vi "ADI_IMU_ADIS16448_AHRS_RoboBees.vi"(8 "Yaw Axis":enum16{"X", "Y", "Z"}(ring)=enum."Z", 9 "Delta t":dbl, 10 "IMU Rates":dbl[](array[numeric])) -> (0 "Yaw":dbl(knob) scale=-180.0..180.0, 1 "Roll":dbl(knob) scale=-180.0..180.0, 2 "Pitch":dbl(knob) scale=-90.0..90.0, 3 "Output":cluster{"Pitch":dbl, "Roll":dbl, "Yaw":dbl})   [LabVIEW 2018, in "ADIS16448_IMU.lvlib"]
uses:
  ADIS16448_IMU.lvlib
panel:
  in  "Tilt Comp (Yaw)":bool=TRUE
  in  "tau mag":dbl=0.04
  in  "tau acc":dbl=0.95
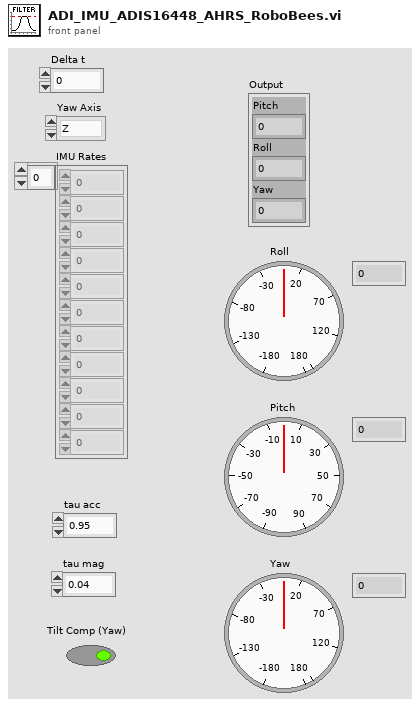
[diagram p1: front panel]
types:
  T1 = cluster{"Xaccel":dbl, "Yaccel":dbl, "Zaccel":dbl}
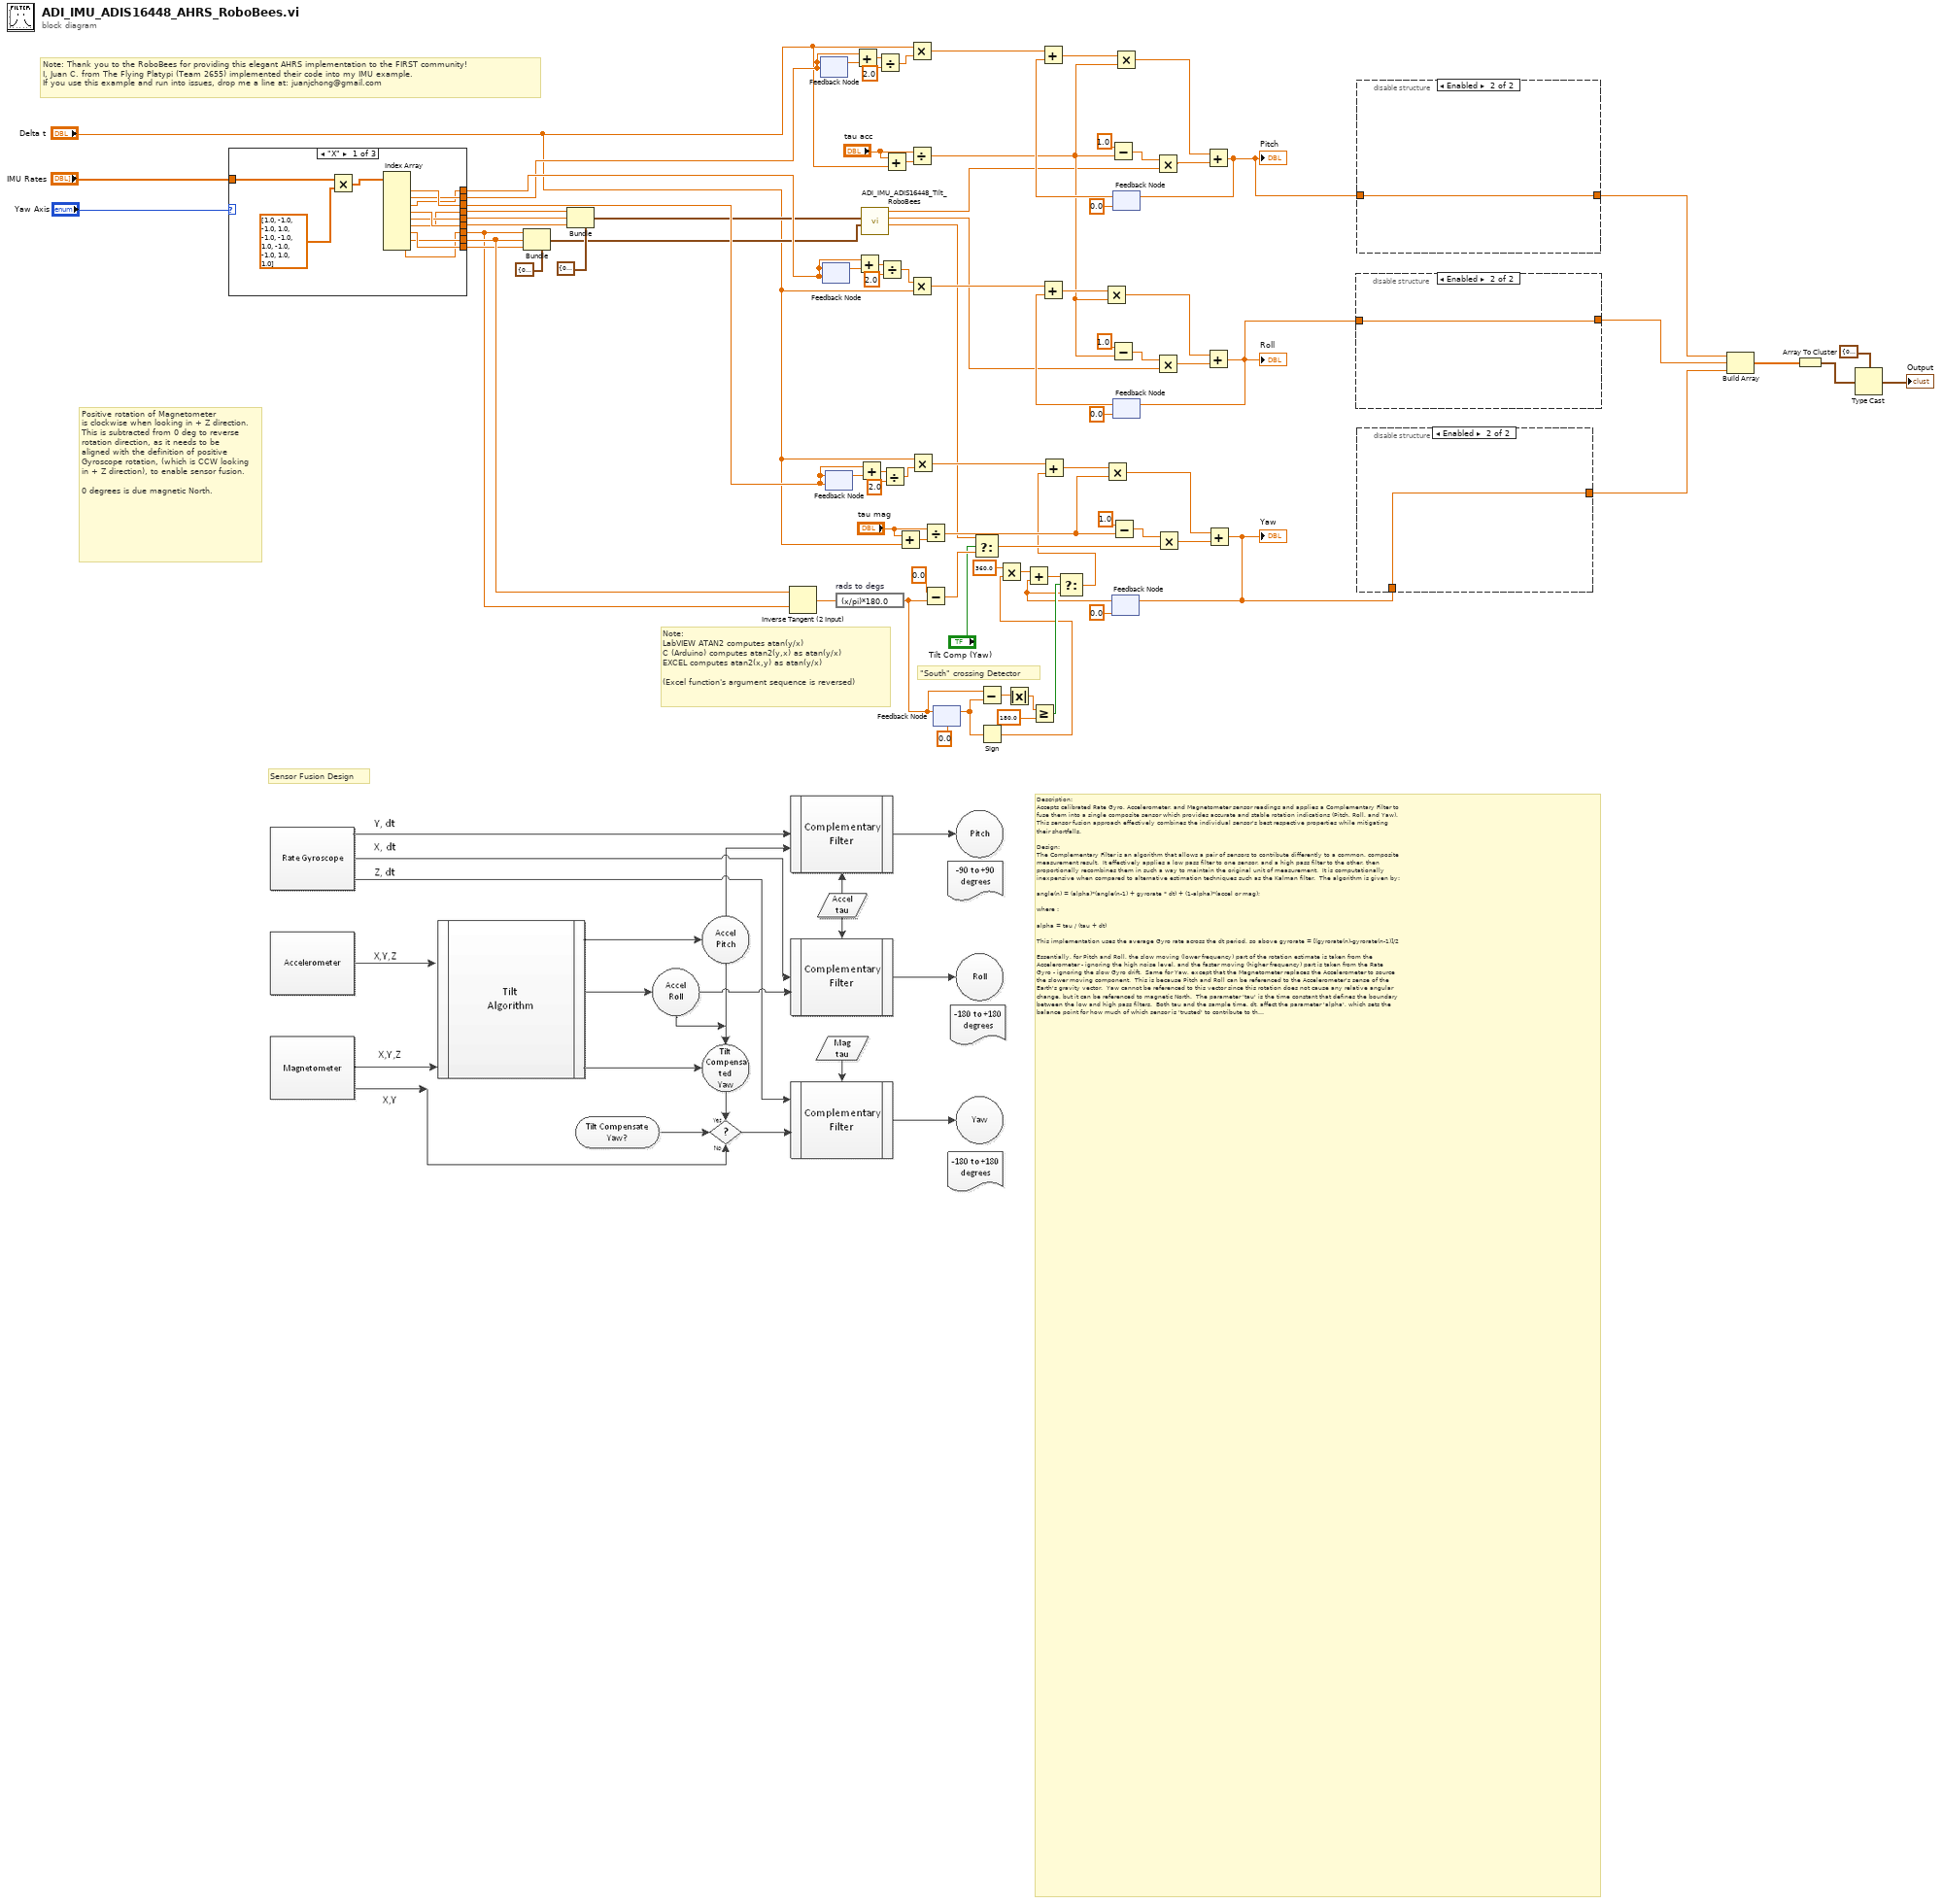
[diagram p0: block diagram]
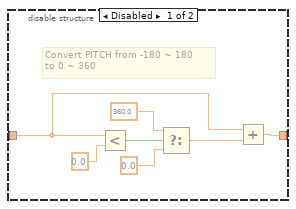
[diagram p2: hidden frame]
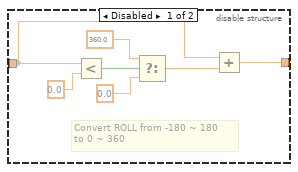
[diagram p3: hidden frame]
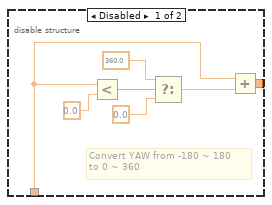
[diagram p4: hidden frame]
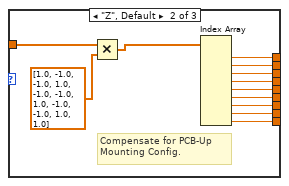
[diagram p5: hidden frame]
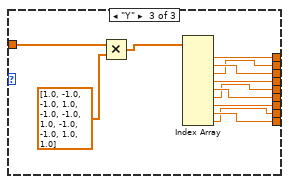
[diagram p6: hidden frame]
diagram:
  # "Note: Thank you to the RoboBees for providing this elegant AHRS implementation to the FIRST community!\nI, Juan C. from The Flying Platypi (Team 2655) implemented their code into my IMU example.\nIf you use this example and run into issues, drop me a line at: juanjchong@gmail.com"
  # "Sensor Fusion Design"
  # "Description:\nAccepts calibrated Rate Gyro, Accelerometer, and Magnetometer sensor readings and applies a Complementary Filter to\nfuse them into a single composite sensor which provides accurate and stable rotation indications (Pitch, Roll, and Yaw).\nThis sensor fusion approach effectively combines the individual sensor's best respective properties while mitigating\ntheir shortfalls.\n\nDesign:\nThe Complementary Filter is an algorithm that allows a pair of sensors to contribute differently to a common, composite\nmeasurement result.  It effectively applies a low pass filter to one sensor, and a high pass filter to the other, then\nproportionally recombines them in such a way to maintain the original unit of measurement.  It is computationally\ninexpensive when compared to alternative estimation techniques such as the Kalman filter.  The algorithm is given by:\n\nangle(n) = (alpha)*(angle(n-1) + gyrorate * dt) + (1-alpha)*(accel or mag);\n\nwhere : \n\nalpha = tau / (tau + dt)\n\nThis implementation uses the average Gyro rate across the dt period, so above gyrorate = [(gyrorate(n)-gyrorate(n-1)]/2\n\nEssentially, for Pitch and Roll, the slow moving (lower frequency) part of the rotation estimate is taken from the\nAccelerometer - ignoring the high noise level, and the faster moving (higher frequency) part is taken from the Rate \nGyro - ignoring the slow Gyro drift.  Same for Yaw, except that the Magnetometer replaces the Accelerometer to source\nthe slower moving component.  This is because Pitch and Roll can be referenced to the Accelerometer's sense of the\nEarth's gravity vector.  Yaw cannot be referenced to this vector since this rotation does not cause any relative angular\nchange, but it can be referenced to magnetic North.  The parameter 'tau' is the time constant that defines the boundary\nbetween the low and high pass filters.  Both tau and the sample time, dt, affect the parameter 'alpha', which sets the\nbalance point for how much of which sensor is 'trusted' to contribute to the rotation estimate.\n\nThe Complementary Filter algorithm is applied to each X/Y/Z rotation axis to compute R/P/Y outputs, respectively.\n\nMagnetometer readings are tilt-compensated when Tilt-Comp-(Yaw) is asserted (True), by the IMU TILT subVI.  This\ncreates what is known as a tilt-compensated compass, which allows Yaw to be insensitive to the effects of a\nnon-level sensor, but generates error in Yaw during movement (coordinate acceleration).\n\nThe Yaw \"South\" crossing detector is necessary to allow a smooth transition across the +/- 180 deg discontinuity (inherent\nin the ATAN function).  Since -180 deg is congruent with +180 deg, Yaw needs to jump between these values when\ncrossing South (North is 0 deg).  The design depends upon comparison of successive Yaw readings to detect a cross-over\nevent.  The cross-over detector monitors the current reading and evaluates how far it is from the previous reading.  If it\nis greater than the previous reading by the Discriminant (= 180 deg), then Yaw just crossed South.\n\nBy choosing 180 as the Discriminant, the only way the detector can produce a false positive, assuming a loop iteration\nof 70 msec, is for it to rotate >2,571 dps ... (2,571=180/.07).  This is faster than the ST L3GD20 Gyro can register.  The\ndetector produces a Boolean True upon detecting a South crossing.  This is used to alter the (n-1) Yaw which was\npreviously stored, either adding or subtracting 360 degrees as required to place the previous Yaw in the correct quadrant\nwhenever crossing occurs.  The Modulus function cannot be used here as the Complementary Filter algorithm has 'state'\n(needs to remember previous Yaw).\n \nWe are in effect stitching together two ends of a ruler for 'modular arithmetic' (clock math).\n\nInputs:\nGYRO - Gyro rate and sample time measurements.\nACCEL - Acceleration measurements.\nMAG - Magnetic measurements.\nTAU ACC - tau parameter used to set sensor balance between Accel and Gyro for Roll and Pitch.\nTAU MAG -  tau parameter used to set sensor balance between Mag and Gyro for Yaw.\nTILT COMP (Yaw) - Enables Yaw tilt-compensation if True.\n\nOutputs:\nROLL - Filtered Roll about sensor X-axis.\nPITCH - Filtered Pitch about sensor Y-axis.\nYAW - Filtered Yaw about sensor Z-axis.\n\nVI Properties:\nExecution Reentrancy is set to Non Reentrant Execution\n\nImplementation:\nIt's best to establish the optimum loop sample time first.  See IMU READ implementation notes for guidance.  Each\ntau parameter should then be adjusted to achieve optimum sensor fusion.  tau acc affects Roll and Pitch, tau mag affects\nYaw.  Start at value 1 or 2 and decrease by half each time until the result doesn't drift, but not so far that the result gets\nnoisy.  An optimum tau for this IMU is likely in the range of 1.0 to 0.01, for a loop sample time between 10 and 100 ms.\n\nNote that both sample timing (dt) and tau both affect the balance parameter, 'alpha'.  Adjusting either dt or tau will\nrequire the other to be readjusted to maintain a particular filter performance.\n\nIt is likely best to set Yaw tilt-compensation to off (False) if the Yaw value is to be used as feedback in a closed loop\ncontrol application.  The tradeoff is that Yaw will only be accurate while the robot is level.\n\nSince a Yaw of -180 degrees is congruent with +180 degrees (they represent the same direction), it is possible that the\nYaw output will oscillate between these two values when the sensor happens to be pointing due South, as sensor\nnoise causes slight variation.  You will need to account for this possibility if you are using the Yaw value for decision-\nmaking in code.\n\n----- The RoboBees FRC Team 836! -----  Complement your passion to solve problems with a STEM Education!"
  # "\"South\" crossing Detector"
  # "Positive rotation of Magnetometer\nis clockwise when looking in + Z direction.  This is subtracted from 0 deg to reverse rotation direction, as it needs to be aligned with the definition of positive Gyroscope rotation, (which is CCW looking in + Z direction), to enable sensor fusion.\n\n0 degrees is due magnetic North."
  # "Note:\nLabVIEW ATAN2 computes atan(y/x)\nC (Arduino) computes atan2(y,x) as atan(y/x)\nEXCEL computes atan2(x,y) as atan(y/x)\n\n(Excel function's argument sequence is reversed)"
  n1 = case shown="\"X\"" "Yaw Axis" {
    tunnel: [w98 w112 w124] -> w28
    tunnel: [w95 w111 w121] -> w21
    tunnel: "IMU Rates" -> [w91 w103 w115]
    tunnel: [w92 w110 w118] -> w23
    tunnel: [w96 w109 w119] -> w20
    tunnel: [w97 w108 w120] -> w19
    tunnel: [w99 w107 w122] -> w27
    tunnel: [w100 w106 w123] -> w26
    tunnel: [w93 w105 w116] -> w25
    tunnel: [w94 w104 w117] -> w24
    frame "X" {
      n2 = Multiply(x=w91, y=dbl[] [1.0, -1.0, -1.0, 1.0, -1.0, -1.0, 1.0, -1.0, -1.0, 1.0, 1.0]) -> (x*y=w90:dbl[])
      n3 = Index Array(array=w90) -> (element #1=w100:dbl, element #2=w99:dbl, element #3=w98:dbl, element #4=w97:dbl, element #5=w96:dbl, element #6=w95:dbl, element #7=w94:dbl, element #8=w93:dbl, element #9=w92:dbl)  [unwired: 9 in]
    }
    frame "Z", Default {
      # "Compensate for PCB-Up\nMounting Config."
      n4 = Multiply(x=w103, y=dbl[] [1.0, -1.0, -1.0, 1.0, -1.0, -1.0, 1.0, -1.0, -1.0, 1.0, 1.0]) -> (x*y=w101:dbl[])
      n5 = Index Array(array=w101) -> (element #1=w112:dbl, element #2=w107:dbl, element #3=w106:dbl, element #4=w111:dbl, element #5=w109:dbl, element #6=w108:dbl, element #7=w110:dbl, element #8=w105:dbl, element #9=w104:dbl)  [unwired: 9 in]
    }
    frame "Y" {
      n6 = Multiply(x=w115, y=dbl[] [1.0, -1.0, -1.0, 1.0, -1.0, -1.0, 1.0, -1.0, -1.0, 1.0, 1.0]) -> (x*y=w113:dbl[])
      n7 = Index Array(array=w113) -> (element #1=w124:dbl, element #2=w123:dbl, element #3=w122:dbl, element #4=w121:dbl, element #5=w120:dbl, element #6=w119:dbl, element #7=w118:dbl, element #8=w117:dbl, element #9=w116:dbl)  [unwired: 9 in]
    }
  }
  n8 = Bundle(cluster=cluster{"Xmag":dbl, "Ymag":dbl, "Zmag":dbl} {"Xmag"=0.0, "Ymag"=0.0, "Zmag"=0.0} ("Mag"), "Xmag"=w23, "Ymag"=w25, "Zmag"=w24) -> (w16:cluster{"Xmag":dbl, "Ymag":dbl, "Zmag":dbl})
  n9 = Bundle(cluster=T1 {"Xaccel"=0.0, "Yaccel"=0.0, "Zaccel"=0.0} ("Accel"), "Xaccel"=w21, "Yaccel"=w20, "Zaccel"=w19) -> (w17:T1)
  n10 = Inverse Tangent (2 Input)(1:w23, 2:w25) -> (0:w61:dbl)
  n11 = feedback #1(w27) -> (w50:dbl)
  n12 = feedback-in #1(w27) -> ()
  n13 = feedback #2(w28) -> (w44:dbl)
  n14 = feedback-in #2(w28) -> ()
  n15 = feedback #3(w26) -> (w42:dbl)
  n16 = feedback-in #3(w26) -> ()
  n17 = expression code="(x/pi)*180.0" "rads to degs"(w61) -> (w31:dbl)
  n18 = Add(x=w27, y=w50) -> (x+y=w49:dbl)
  n19 = Add(x=w28, y=w44) -> (x+y=w45:dbl)
  n20 = Add(x=w26, y=w42) -> (x+y=w41:dbl)
  n21 = call "ADI_IMU_ADIS16448_Tilt_RoboBees.vi"("Mag"=w16, "Accel"=w17) -> ("Yaw"=w13:dbl, "Roll"=w14:dbl, "Pitch"=w15:dbl)  [unwired: 6 in, 1 out]
  n22 = Divide(x=w49, y=2.0) -> (x/y=w47:dbl)
  n23 = Divide(x=w45, y=2.0) -> (x/y=w43:dbl)
  n24 = Divide(x=w41, y=2.0) -> (x/y=w39:dbl)
  n25 = Add(x="tau acc", y="Delta t") -> (x+y=w87:dbl)
  n26 = Add(x="tau mag", y="Delta t") -> (x+y=w62:dbl)
  n27 = Multiply(x="Delta t", y=w47) -> (x*y=w75:dbl)
  n28 = Divide(x="tau acc", y=w87) -> (x/y=w71:dbl)
  n29 = Multiply(x=w43, y="Delta t") -> (x*y=w85:dbl)
  n30 = Multiply(x="Delta t", y=w39) -> (x*y=w55:dbl)
  n31 = Divide(x="tau mag", y=w62) -> (x/y=w54:dbl)
  n32 = Subtract(x=0.0 ("y"), y=w31) -> (x-y=w58:dbl)
  n33 = feedback #4(0.0) -> (w32:dbl)
  n34 = feedback-in #4(w31) -> ()
  n35 = Select(t=w13, s="Tilt Comp (Yaw)", f=w58) -> (s? t:f=w59:dbl)
  n36 = Subtract(x=w31, y=w32) -> (x-y=w38:dbl)
  n37 = Sign(1:w32) -> (0:w34:dbl)
  n38 = Multiply(x=360.0 ("y"), y=w34) -> (x*y=w30:dbl)
  n39 = Absolute Value(x=w38) -> (abs(x)=w37:dbl)
  n40 = Greater Or Equal?(x=w37, y=180.0) -> (x >= y?=w35:bool)
  n41 = Subtract(x=1.0, y=w71) -> (x-y=w74:dbl)
  n42 = Subtract(x=1.0, y=w71) -> (x-y=w70:dbl)
  n43 = Subtract(x=1.0, y=w54) -> (x-y=w68:dbl)
  n44 = feedback #5(0.0) -> (w29:dbl)
  n45 = Add(x=w30, y=w29) -> (x+y=w51:dbl)
  n46 = Select(t=w51, s=w35, f=w29) -> (s? t:f=w52:dbl)
  n47 = Add(x=w55, y=w52) -> (x+y=w65:dbl)
  n48 = Multiply(x=w65, y=w54) -> (x*y=w67:dbl)
  n49 = feedback #6(0.0) -> (w79:dbl)
  n50 = Add(x=w75, y=w79) -> (x+y=w76:dbl)
  n51 = Multiply(x=w76, y=w71) -> (x*y=w78:dbl)
  n52 = feedback #7(0.0) -> (w69:dbl)
  n53 = Add(x=w85, y=w69) -> (x+y=w84:dbl)
  n54 = Multiply(x=w84, y=w71) -> (x*y=w82:dbl)
  n55 = Multiply(x=w74, y=w15) -> (x*y=w77:dbl)
  n56 = Multiply(x=w70, y=w14) -> (x*y=w83:dbl)
  n57 = Multiply(x=w68, y=w59) -> (x*y=w66:dbl)
  n58 = Add(x=w78, y=w77) -> (x+y=w3:dbl)
  "Pitch" <- w3
  n59 = feedback-in #6(w3) -> ()
  n60 = Add(x=w82, y=w83) -> (x+y=w2:dbl)
  "Roll" <- w2
  n61 = feedback-in #7(w2) -> ()
  n62 = Add(x=w67, y=w66) -> (x+y=w12:dbl)
  "Yaw" <- w12
  n63 = feedback-in #5(w12) -> ()
  n64 = disable-structure shown="Enabled" {
    disable-tunnel: w2 -> [w126 w132]
    disable-tunnel: [w125 w132] -> w10
    frame Disabled {
      # "Convert ROLL from -180 ~ 180 \nto 0 ~ 360"
      n65 = Less?(x=w126, y=0.0) -> (x < y?=w130:bool)
      n66 = Select(t=360.0, s=w130, f=0.0) -> (s? t:f=w127:dbl)
      n67 = Add(x=w126, y=w127) -> (x+y=w125:dbl)
    }
    frame Enabled {
    }
  }
  n68 = disable-structure shown="Enabled" {
    disable-tunnel: [w134 w140] -> w9
    disable-tunnel: w3 -> [w133 w140]
    frame Disabled {
      # "Convert PITCH from -180 ~ 180 \nto 0 ~ 360"
      n69 = Less?(x=w133, y=0.0) -> (x < y?=w138:bool)
      n70 = Select(t=360.0, s=w138, f=0.0) -> (s? t:f=w135:dbl)
      n71 = Add(x=w133, y=w135) -> (x+y=w134:dbl)
    }
    frame Enabled {
    }
  }
  n72 = disable-structure shown="Enabled" {
    disable-tunnel: w12 -> [w142 w148]
    disable-tunnel: [w141 w148] -> w11
    frame Disabled {
      # "Convert YAW from -180 ~ 180 \nto 0 ~ 360"
      n73 = Less?(x=w142, y=0.0) -> (x < y?=w146:bool)
      n74 = Select(t=360.0, s=w146, f=0.0) -> (s? t:f=w143:dbl)
      n75 = Add(x=w142, y=w143) -> (x+y=w141:dbl)
    }
    frame Enabled {
    }
  }
  n76 = Build Array(w9, w10, w11) -> (w5:dbl[])
  n77 = Array To Cluster(array=w5) -> (cluster=w6:cluster{"[0]":dbl, "[1]":dbl, "[2]":dbl})
  n78 = Type Cast(type=cluster{"Pitch":dbl, "Roll":dbl, "Yaw":dbl} {"Pitch"=0.0, "Roll"=0.0, "Yaw"=0.0} ("IMU AHRS"), x=w6) -> (*(type *) &x=→"Output":cluster{"Pitch":dbl, "Roll":dbl, "Yaw":dbl})
